vi "DSF.Engine.Buffer Converter.Build.vi"(8 "error in (no error)":errorcluster, 9 "channel blocks":T1[](array[typedef]) {"count" format="%d elements"; "First Channel Descriptor"."base address" format="%016x"; "First Channel Descriptor"."Channel Parameters"."offset" format="%d bytes"}, 10 "Buffer in":refnum<class "DSF.Engine.Memory.Buffer.lvclass">, 11 "Buffer Converter in":refnum<class "Buffer Converter.lvclass">) -> (0 "error out":errorcluster, 2 "Buffer out":refnum<class "DSF.Engine.Memory.Buffer.lvclass">, 3 "Buffer Converter out":refnum<class "Buffer Converter.lvclass">)   [LabVIEW 2017, in "DSF.Engine.lvlib" / "Buffer Converter.lvclass"]
uses:
  Buffer Converter.lvclass
  DSF.Engine.Memory.Buffer.lvclass
  Shared/Typedefs/DSF.Shared.Typedefs.Configuration.Transfer.Channel Block Descriptor.ctl
  Shared/Typedefs/DSF.Shared.Typedefs.Configuration.Transfer.Channel Descriptor.ctl
  Shared/Typedefs/DSF.Shared.Typedefs.Configuration.Transfer.Channel Parameters.ctl
  Shared/Typedefs/DSF.Shared.Typedefs.Data Type.ctl
  Buffer Converter.lvclass/Buffer Converter.ctl
  DSF.Engine.Memory.Buffer.Write.1D.Bool.vi
  DSF.Engine.Memory.Buffer.Write.1D.SGL.vi
  DSF.Engine.Memory.Buffer.Write.1D.DBL.vi
  DSF.Engine.Memory.Buffer.Write.1D.I8.vi
  DSF.Engine.Memory.Buffer.Write.1D.I16.vi
  DSF.Engine.Memory.Buffer.Write.1D.I32.vi
  DSF.Engine.Memory.Buffer.Write.1D.I64.vi
  DSF.Engine.Memory.Buffer.Write.1D.U8.vi
  DSF.Engine.Memory.Buffer.Write.1D.U16.vi
  DSF.Engine.Memory.Buffer.Write.1D.U32.vi
  DSF.Engine.Memory.Buffer.Write.1D.U64.vi
  DSF.Engine.lvlib
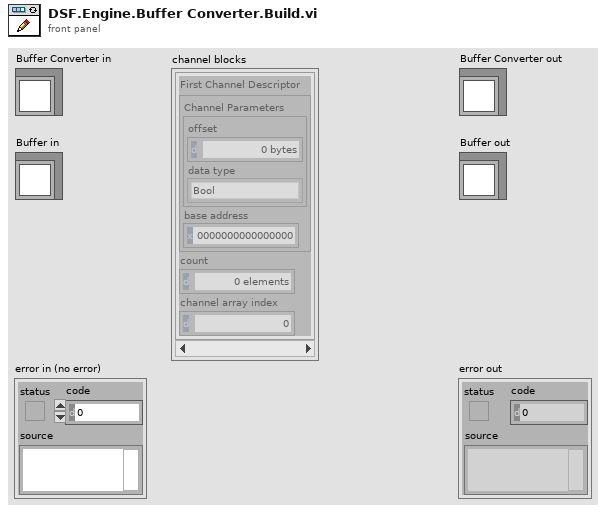
[diagram p1: front panel]
types:
  T1 = typedef "DSF.Engine.lvlib/DSF.Shared.Typedefs.Configuration.Transfer.Channel Block Descriptor.ctl" = cluster{"First Channel Descriptor":T2, "count":u64, "channel array index":u64}
  T2 = typedef "DSF.Engine.lvlib/DSF.Shared.Typedefs.Configuration.Transfer.Channel Descriptor.ctl" = cluster{"Channel Parameters":T3, "base address":u64}
  T3 = typedef "DSF.Engine.lvlib/DSF.Shared.Typedefs.Configuration.Transfer.Channel Parameters.ctl" = cluster{"offset":u64, "data type":T4}
  T4 = typedef "DSF.Engine.lvlib/DSF.Shared.Typedefs.Data Type.ctl" = enum8{"Bool", "SGL", "DBL", "I8", "I16", "I32", "I64", "U8", "U16", "U32", "U64"}
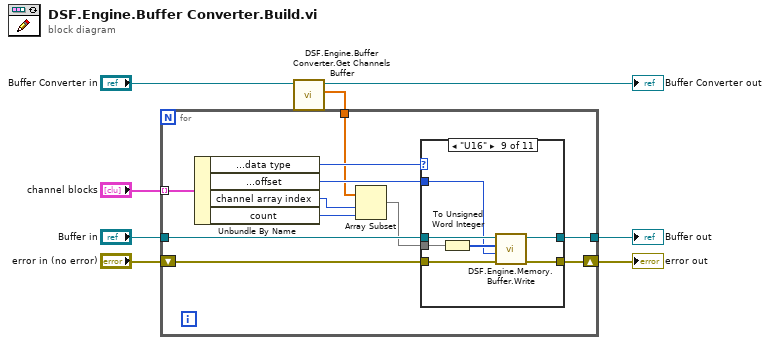
[diagram p0: block diagram]
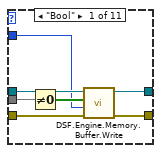
[diagram p2: hidden frame]
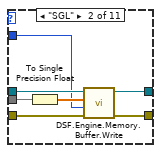
[diagram p3: hidden frame]
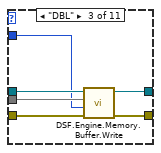
[diagram p4: hidden frame]
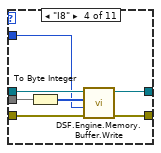
[diagram p5: hidden frame]
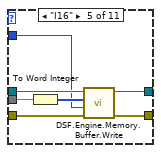
[diagram p6: hidden frame]
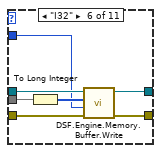
[diagram p7: hidden frame]
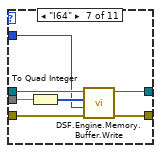
[diagram p8: hidden frame]
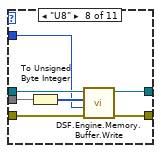
[diagram p9: hidden frame]
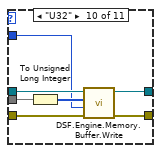
[diagram p10: hidden frame]
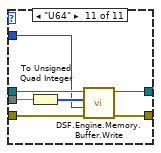
[diagram p11: hidden frame]
diagram:
  n1 = call "DSF.Engine.Buffer Converter.Get Channels Buffer.vi"("Buffer Converter in"="Buffer Converter in") -> ("channels buffer"=w2:dbl[], "Buffer Converter out"=→"Buffer Converter out":refnum<class "Buffer Converter.lvclass">)  [unwired: 9 in]
  n2 = for {
    tunnel: "channel blocks" -> [w12] mode=indexing
    tunnel: w2 -> [w9]
    shift-right: [w10] -> w3
    shift-left: "error in (no error)" -> [w11]
    tunnel: "Buffer in" -> [w15]
    tunnel: [w14] -> w7
    n3 = Unbundle By Name(w12) -> ("First Channel Descriptor.Channel Parameters.data type"=w16:T4, "First Channel Descriptor.Channel Parameters.offset"=w19:u64, "channel array index"=w18:u64, "count"=w17:u64)
    n4 = Array Subset(array=w9, index=w18, length=w17) -> (w13:dbl[])
    n5 = case shown="\"U16\"" w16 {
      tunnel: w15 -> [w26 w33 w39 w46 w53 w60 w67 w74 w81 w88 w95]
      tunnel: w13 -> [w21 w28 w35 w41 w48 w55 w62 w69 w76 w83 w90]
      tunnel: w11 -> [w25 w32 w38 w45 w52 w59 w66 w73 w80 w87 w94]
      tunnel: [w24 w31 w37 w44 w51 w58 w65 w72 w79 w86 w93] -> w10
      tunnel: w19 -> [w22 w29 w34 w42 w49 w56 w63 w70 w77 w84 w91]
      tunnel: [w20 w27 w36 w40 w47 w54 w61 w68 w75 w82 w89] -> w14
      frame "Bool" {
        n6 = Not Equal To 0?(x=w21) -> (x != 0?=w23:bool[])
        n7 = call-poly "DSF.Engine.Memory.Buffer.Write.vi"("error in (no error)"=w25, "offset (0)"=w22, "buffer in"=w23, "Buffer in"=w26) -> ("error out"=w24:errorcluster, "Buffer out"=w20:refnum<class "DSF.Engine.Memory.Buffer.lvclass">)  [unwired: 4 in, 2 out]
      }
      frame "SGL" {
        n8 = To Single Precision Float(number=w28) -> (single precision float=w30:sgl[])
        n9 = call-poly "DSF.Engine.Memory.Buffer.Write.vi"("error in (no error)"=w32, "offset (0)"=w29, "buffer in"=w30, "Buffer in"=w33) -> ("error out"=w31:errorcluster, "Buffer out"=w27:refnum<class "DSF.Engine.Memory.Buffer.lvclass">)  [unwired: 4 in, 2 out]
      }
      frame "DBL" {
        n10 = call-poly "DSF.Engine.Memory.Buffer.Write.vi"("error in (no error)"=w38, "offset (0)"=w34, "buffer in"=w35, "Buffer in"=w39) -> ("error out"=w37:errorcluster, "Buffer out"=w36:refnum<class "DSF.Engine.Memory.Buffer.lvclass">)  [unwired: 4 in, 2 out]
      }
      frame "I8" {
        n11 = To Byte Integer(number=w41) -> (8bit integer=w43:i8[])
        n12 = call-poly "DSF.Engine.Memory.Buffer.Write.vi"("error in (no error)"=w45, "offset (0)"=w42, "buffer in"=w43, "Buffer in"=w46) -> ("error out"=w44:errorcluster, "Buffer out"=w40:refnum<class "DSF.Engine.Memory.Buffer.lvclass">)  [unwired: 4 in, 2 out]
      }
      frame "I16" {
        n13 = To Word Integer(number=w48) -> (16bit integer=w50:i16[])
        n14 = call-poly "DSF.Engine.Memory.Buffer.Write.vi"("error in (no error)"=w52, "offset (0)"=w49, "buffer in"=w50, "Buffer in"=w53) -> ("error out"=w51:errorcluster, "Buffer out"=w47:refnum<class "DSF.Engine.Memory.Buffer.lvclass">)  [unwired: 4 in, 2 out]
      }
      frame "I32" {
        n15 = To Long Integer(number=w55) -> (32bit integer=w57:i32[])
        n16 = call-poly "DSF.Engine.Memory.Buffer.Write.vi"("error in (no error)"=w59, "offset (0)"=w56, "buffer in"=w57, "Buffer in"=w60) -> ("error out"=w58:errorcluster, "Buffer out"=w54:refnum<class "DSF.Engine.Memory.Buffer.lvclass">)  [unwired: 4 in, 2 out]
      }
      frame "I64" {
        n17 = To Quad Integer(1:w62) -> (0:w64:i64[])
        n18 = call-poly "DSF.Engine.Memory.Buffer.Write.vi"("error in (no error)"=w66, "offset (0)"=w63, "buffer in"=w64, "Buffer in"=w67) -> ("error out"=w65:errorcluster, "Buffer out"=w61:refnum<class "DSF.Engine.Memory.Buffer.lvclass">)  [unwired: 4 in, 2 out]
      }
      frame "U8" {
        n19 = To Unsigned Byte Integer(number=w69) -> (unsigned 8bit integer=w71:u8[])
        n20 = call-poly "DSF.Engine.Memory.Buffer.Write.vi"("error in (no error)"=w73, "offset (0)"=w70, "buffer in"=w71, "Buffer in"=w74) -> ("error out"=w72:errorcluster, "Buffer out"=w68:refnum<class "DSF.Engine.Memory.Buffer.lvclass">)  [unwired: 4 in, 2 out]
      }
      frame "U16" {
        n21 = To Unsigned Word Integer(number=w76) -> (unsigned 16bit integer=w78:u16[])
        n22 = call-poly "DSF.Engine.Memory.Buffer.Write.vi"("error in (no error)"=w80, "offset (0)"=w77, "buffer in"=w78, "Buffer in"=w81) -> ("error out"=w79:errorcluster, "Buffer out"=w75:refnum<class "DSF.Engine.Memory.Buffer.lvclass">)  [unwired: 4 in, 2 out]
      }
      frame "U32" {
        n23 = To Unsigned Long Integer(number=w83) -> (unsigned 32bit integer=w85:u32[])
        n24 = call-poly "DSF.Engine.Memory.Buffer.Write.vi"("error in (no error)"=w87, "offset (0)"=w84, "buffer in"=w85, "Buffer in"=w88) -> ("error out"=w86:errorcluster, "Buffer out"=w82:refnum<class "DSF.Engine.Memory.Buffer.lvclass">)  [unwired: 4 in, 2 out]
      }
      frame "U64" {
        n25 = To Unsigned Quad Integer(1:w90) -> (0:w92:u64[])
        n26 = call-poly "DSF.Engine.Memory.Buffer.Write.vi"("error in (no error)"=w94, "offset (0)"=w91, "buffer in"=w92, "Buffer in"=w95) -> ("error out"=w93:errorcluster, "Buffer out"=w89:refnum<class "DSF.Engine.Memory.Buffer.lvclass">)  [unwired: 4 in, 2 out]
      }
    }
  }
  "error out" <- w3
  "Buffer out" <- w7
